vi "file -- accumulate data files.vi"(11 "list of <mmddyy> folders":path[](array[path])) -> (0 "timestamp array":dbl[](array[numeric]), 2 "sweep file name  array":T1[](array[typedef]))   [LabVIEW 2012]
uses:
  sweep file name.ctl
  find all matching strings in the list.vi
  Split file name.vi
panel:
  in  "sweep file name":T1={"temperature"=0.0, "temperature str"="", "file path"=path "/snowfall/Users/arcadi/Desktop/Ultrasound/Experiment/YBCO_4/Round1/Sweep12/June_2011/062511/221.16400K_300_3100_001_062511.dat", "last mod"=timestamp(0 s since 1904-01-01), "file name str"="", "mod time(min)"=0.0, "file format"=enum.""}
  in  "dummy":T1={"temperature"=0.0, "temperature str"="", "file path"=path "/snowfall/Users/arcadi/Desktop/Ultrasound/Experiment/YBCO_4/Round1/Sweep12/June_2011/062511/221.16400K_300_3100_001_062511.dat", "last mod"=timestamp(0 s since 1904-01-01), "file name str"="", "mod time(min)"=0.0, "file format"=enum.""}
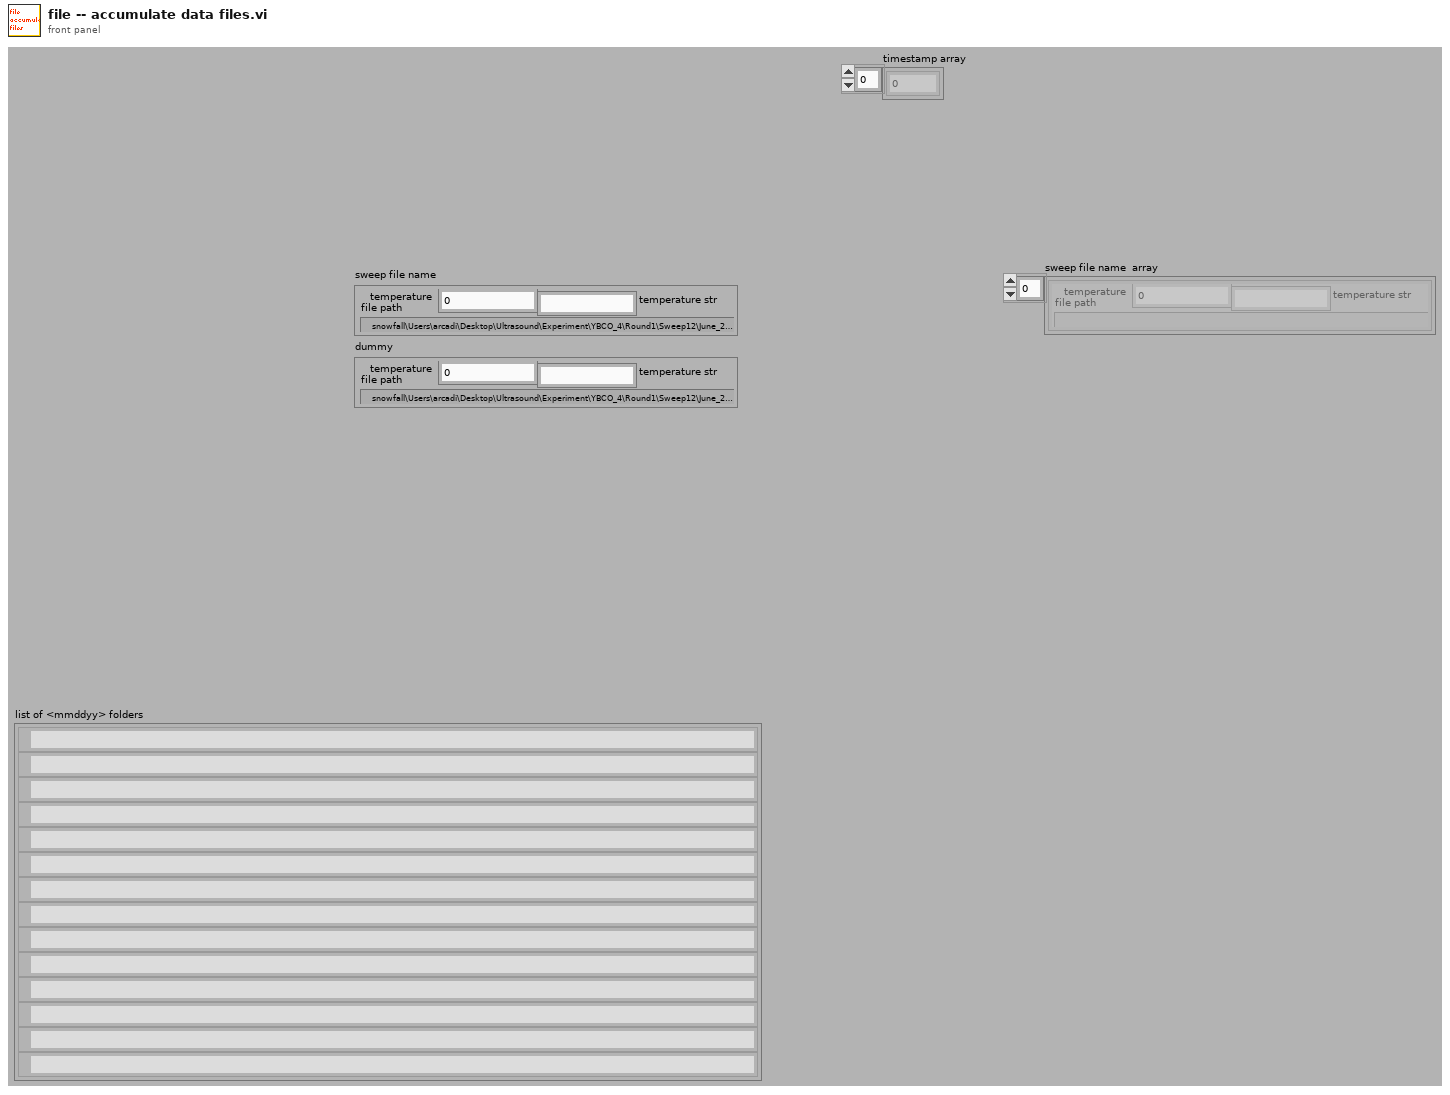
[diagram p1: front panel]
types:
  T1 = typedef "sweep file name.ctl" = cluster{"temperature":dbl, "temperature str":string, "file path":path, "last mod":timestamp, "file name str":string, "mod time(min)":dbl, "file format":enum16{"", "ascii", "binary"}}
  T2 = cluster{"basename":string, "dat":bool, "bin":bool}[]
  T3 = cluster{"temperature":string, "from F":string, "to F":string, "counter":string, "date":string}
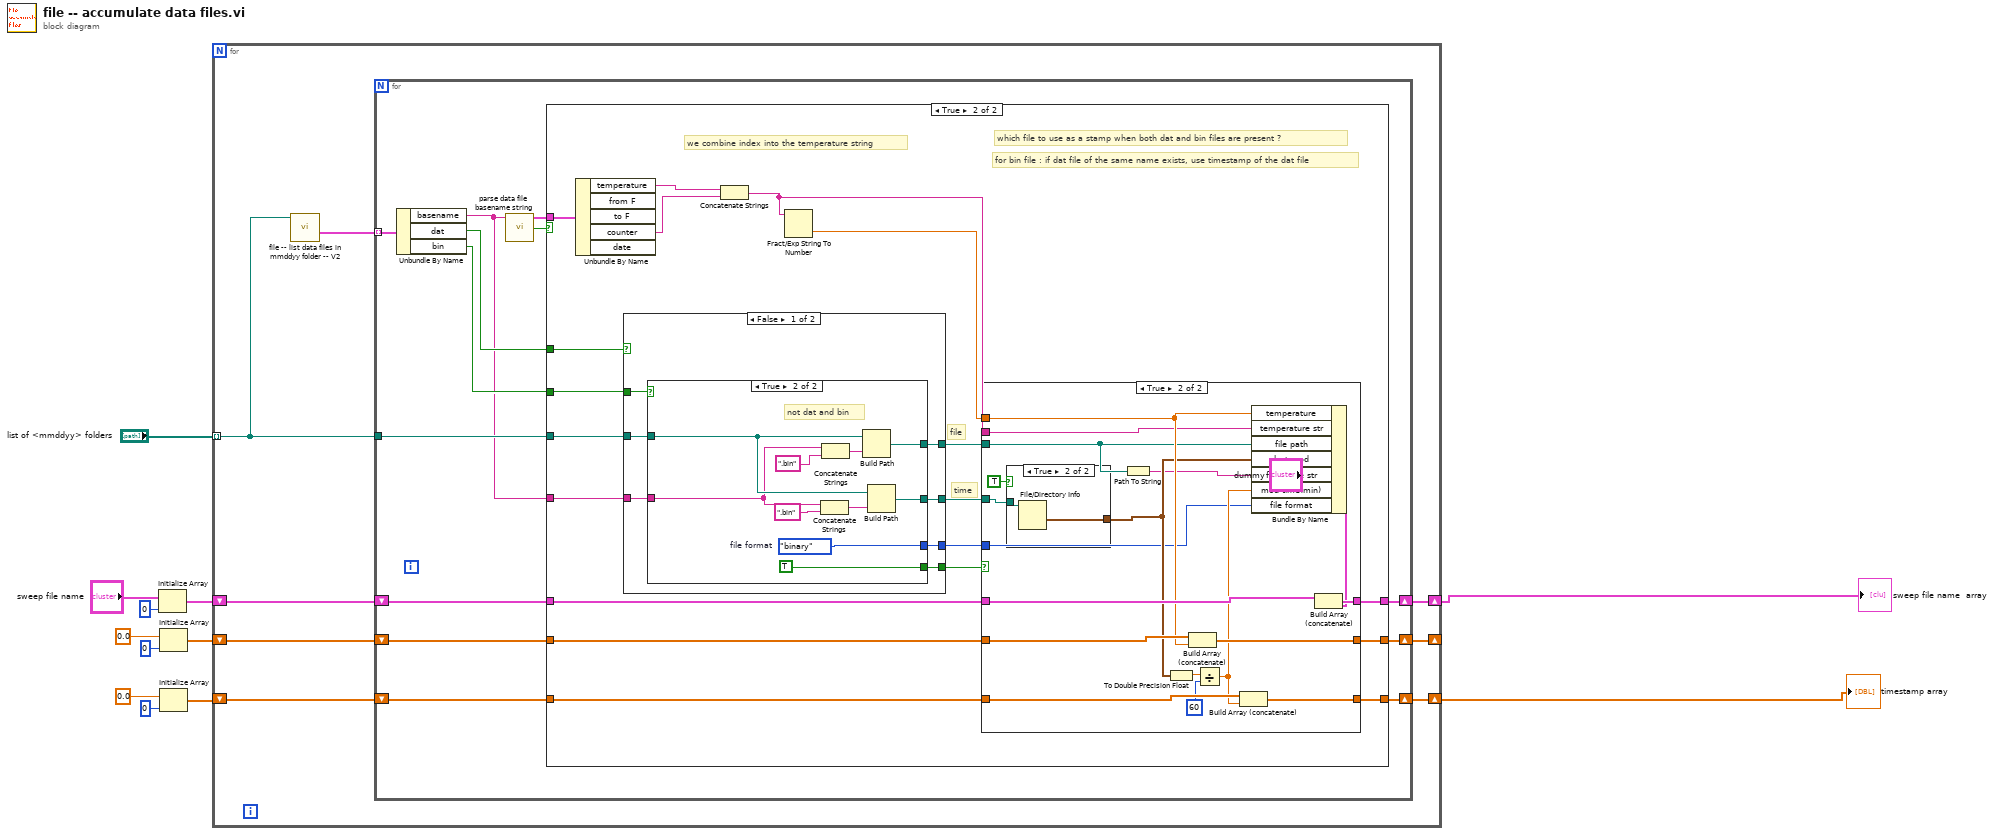
[diagram p0: block diagram]
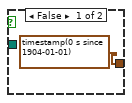
[diagram p4: hidden frame]
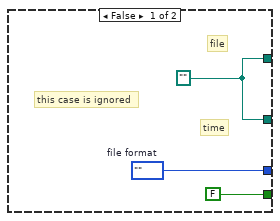
[diagram p5: hidden frame]
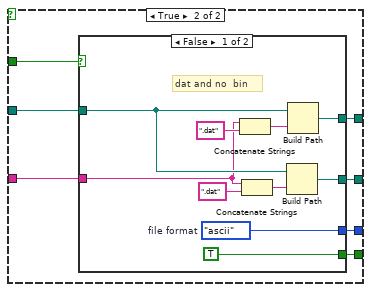
[diagram p6: hidden frame]
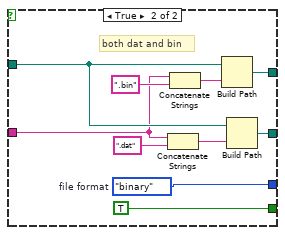
[diagram p7: hidden frame]
diagram:
  n1 = Initialize Array("sweep file name", 0 ("dimension size")) -> (w5:T1[])
  n2 = Initialize Array(0.0 ("dimension size"), 0 ("dimension size")) -> (w4:dbl[])
  n3 = Initialize Array(0.0 ("dimension size"), 0 ("dimension size")) -> (w3:dbl[])
  n4 = for {
    tunnel: "list of <mmddyy> folders" -> [w13] mode=indexing
    shift-right: [w18] -> w2
    shift-left: w5 -> [w20]
    shift-right: [w19] -> _
    shift-left: w4 -> [w17]
    shift-right: [w15] -> w1
    shift-left: w3 -> [w16]
    n5 = call "file -- list data files in mmddyy folder -- V2.vi"("<mmddyy> folder path"=w13) -> ("Array"=w14:T2)  [unwired: 10 in]
    n6 = for {
      tunnel: w14 -> [w26] mode=indexing
      tunnel: w13 -> [w33]
      shift-right: [w31] -> w18
      shift-left: w20 -> [w32]
      shift-right: [w29] -> w19
      shift-left: w17 -> [w30]
      shift-right: [w27] -> w15
      shift-left: w16 -> [w28]
      n7 = Unbundle By Name(w26) -> ("basename"=w21:string, "dat"=w23:bool, "bin"=w22:bool)
      n8 = call "parse data file basename string.vi"("base name"=w21) -> ("output cluster"=w24:T3, "exact match"=w25:bool)  [unwired: 9 in]
      n9 = case shown="True" w25 {
        tunnel: w33 -> [_ w43]
        tunnel: w32 -> [w36 w55]
        tunnel: [w36 w54] -> w31
        tunnel: w30 -> [w35 w53]
        tunnel: [w35 w52] -> w29
        tunnel: w28 -> [w34 w51]
        tunnel: [w34 w50] -> w27
        tunnel: w24 -> [_ w48]
        tunnel: w23 -> [_ w45]
        tunnel: w22 -> [_ w44]
        tunnel: w21 -> [_ w42]
        frame False {
        }
        frame True {
          # "file"
          # "time"
          # "we combine index into the temperature string"
          # "which file to use as a stamp when both dat and bin files are present ?"
          # "for bin file : if dat file of the same name exists, use timestamp of the dat file"
          n10 = Unbundle By Name(w48) -> ("temperature"=w47:string, "counter"=w46:string)  [unwired: 3 out]
          n11 = case shown="False" w45 {
            tunnel: w44 -> [w82 w107]
            tunnel: w43 -> [w84 w106]
            tunnel: w42 -> [w83 w105]
            tunnel: [w87 w104] -> w39
            tunnel: [w86 w103] -> w41
            tunnel: [w85 w102] -> w40
            tunnel: [w81 w101] -> w37
            frame False {
              n12 = case shown="True" w82 {
                tunnel: w84 -> [_ w96]
                tunnel: w83 -> [_ w95]
                tunnel: [w88 w99] -> w87
                tunnel: [w88 w94] -> w86
                tunnel: [w90 w92] -> w85
                tunnel: [FALSE ("quote specials") TRUE ("quote specials")] -> w81
                frame False {
                  w88 = path ""
                  w90 = enum16{"", "ascii", "binary"}.""  # file format
                  # "time"
                  # "file"
                  # "this case is ignored"
                }
                frame True {
                  w92 = enum16{"", "ascii", "binary"}."binary"  # file format
                  # "not dat and bin"
                  n13 = Concatenate Strings(w95, ".bin" ("string")) -> (w97:string)
                  n14 = Concatenate Strings(w95, ".bin" ("string")) -> (w93:string)
                  n15 = Build Path(base path=w96, name or relative path=w93) -> (appended path=w99:path)
                  n16 = Build Path(base path=w96, name or relative path=w97) -> (appended path=w94:path)
                }
              }
            }
            frame True {
              n17 = case shown="False" w107 {
                tunnel: w106 -> [w113 w123]
                tunnel: w105 -> [w109 w122]
                tunnel: [w112 w126] -> w104
                tunnel: [w111 w121] -> w103
                tunnel: [w110 w119] -> w102
                tunnel: [TRUE ("quote specials") TRUE ("quote specials")] -> w101
                frame False {
                  w110 = enum16{"", "ascii", "binary"}."ascii"  # file format
                  # "dat and no  bin"
                  n18 = Concatenate Strings(w109, ".dat" ("string")) -> (w114:string)
                  n19 = Concatenate Strings(w109, ".dat" ("string")) -> (w115:string)
                  n20 = Build Path(base path=w113, name or relative path=w115) -> (appended path=w111:path)
                  n21 = Build Path(base path=w113, name or relative path=w114) -> (appended path=w112:path)
                }
                frame True {
                  w119 = enum16{"", "ascii", "binary"}."binary"  # file format
                  # "both dat and bin"
                  n22 = Concatenate Strings(w122, ".dat" ("string")) -> (w124:string)
                  n23 = Concatenate Strings(w122, ".bin" ("string")) -> (w120:string)
                  n24 = Build Path(base path=w123, name or relative path=w120) -> (appended path=w126:path)
                  n25 = Build Path(base path=w123, name or relative path=w124) -> (appended path=w121:path)
                }
              }
            }
          }
          n26 = Concatenate Strings(w47, w46) -> (w38:string)
          n27 = Fract/Exp String To Number(string=w38) -> (number=w49:dbl)  [unwired: 3 in, 1 out]
          n28 = case shown="True" w37 {
            tunnel: w55 -> [w58 w77]
            tunnel: [w58 w76] -> w54
            tunnel: w53 -> [w57 w75]
            tunnel: [w57 w74] -> w52
            tunnel: w51 -> [w56 w73]
            tunnel: [w56 w72] -> w50
            tunnel: w49 -> [_ w69]
            tunnel: w41 -> [_ w64]
            tunnel: w40 -> [_ w63]
            tunnel: w39 -> [_ w62]
            tunnel: w38 -> [_ w60]
            frame False {
            }
            frame True {
              n29 = case shown="True" TRUE {
                tunnel: [timestamp(0 s since 1904-01-01) ("last mod") w80] -> w68
                tunnel: w64 -> [_ w79]
                frame False {
                }
                frame True {
                  n30 = File/Directory Info(path=w79) -> (last mod=w80:timestamp)  [unwired: 1 in, 6 out]
                }
              }
              n31 = Path To String(path=w62) -> (string=w61:string)
              n32 = To Double Precision Float(number=w68) -> (double precision float=w67:dbl)
              n33 = Build Array (concatenate)(w75, w69) -> (w74:dbl[])
              n34 = Divide(x=w67, y=60) -> (x/y=w65:dbl)
              n35 = Build Array (concatenate)(w73, w65) -> (w72:dbl[])
              n36 = Bundle By Name(cluster="dummy", "temperature"=w69, "temperature str"=w60, "file path"=w62, "last mod"=w68, "file name str"=w61, "mod time(min)"=w65, "file format"=w63) -> (w70:T1)
              n37 = Build Array (concatenate)(w77, w70) -> (w76:T1[])
            }
          }
        }
      }
    }
  }
  "sweep file name  array" <- w2
  "timestamp array" <- w1
